vi "Send Variant Value.vi"(6 "Name":string, 8 "error in (no error)":errorcluster, 9 "Value":variant, 11 "Message Enqueuer in":refnum<class "Message Enqueuer.lvclass">) -> (0 "error out":errorcluster)   [LabVIEW 2015, in "ActorAutoRegistration.lvlib" / "VariantValueMsg.lvclass"]
uses:
  VariantValueMsg.lvclass
  <vilib>/ActorFramework/Message Enqueuer/Message Enqueuer.lvclass
  VariantValueMsg.lvclass/VariantValueMsg.ctl
  EventDataMessage/EventDataMessage.lvclass
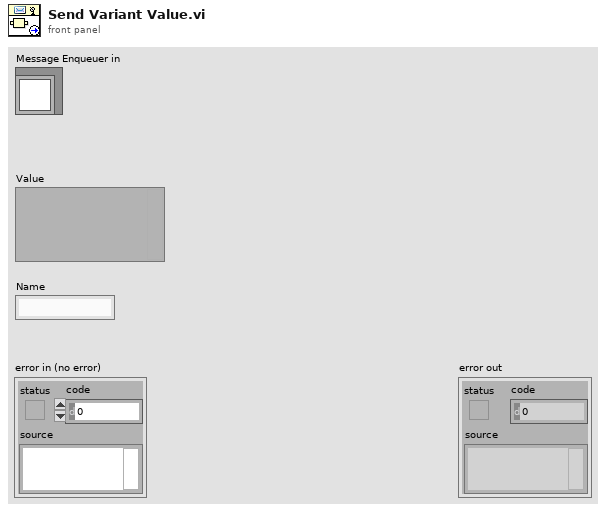
[diagram p1: front panel]
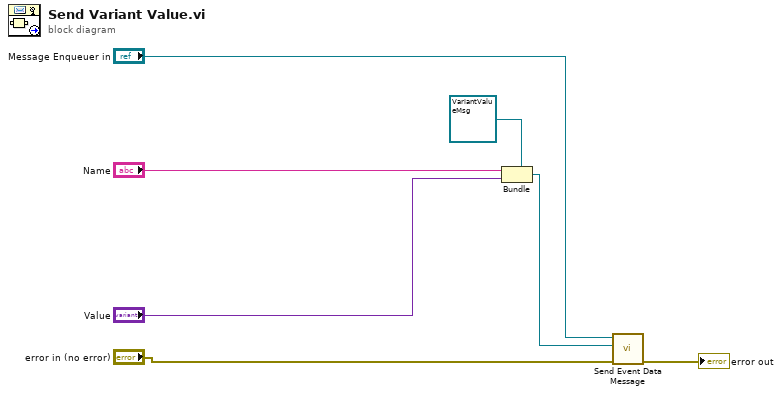
[diagram p0: block diagram]
diagram:
  n1 = Bundle(cluster=refnum<class "VariantValueMsg.lvclass"> refnum ("VariantValueMsg"), "Name", "Value") -> (w3:refnum<class "VariantValueMsg.lvclass">)
  n2 = call "Send Event Data Message.vi"("error in (no error)"="error in (no error)", "EventDataMessage in"=w3, "Message Enqueuer in"="Message Enqueuer in") -> ("error out"=→"error out":errorcluster)  [unwired: 8 in]
